vi "Calculator.vi"() -> ()   [LabVIEW 2014]
panel:
  in  ".":bool
  in  "0":bool
  out "display":string
  in  "=":bool
  in  "plus":bool
  in  "clear":bool
  in  "minus":bool
  in  "3":bool
  in  "2":bool
  in  "1":bool
  in  "multiply":bool
  in  "6":bool
  in  "5":bool
  in  "4":bool
  in  "division":bool
  in  "9":bool
  in  "8":bool
  in  "7":bool
  # "Calculator"
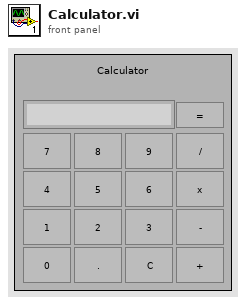
[diagram p1: front panel]
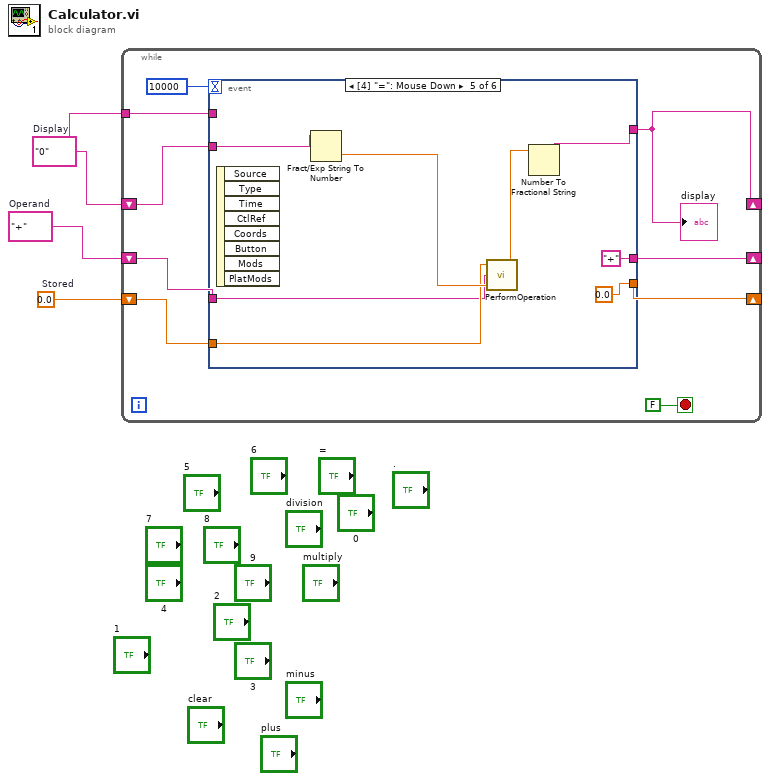
[diagram p0: block diagram]
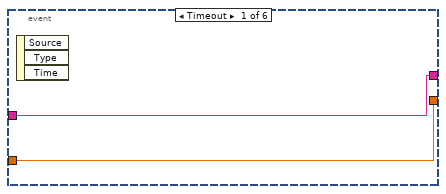
[diagram p2: hidden frame]
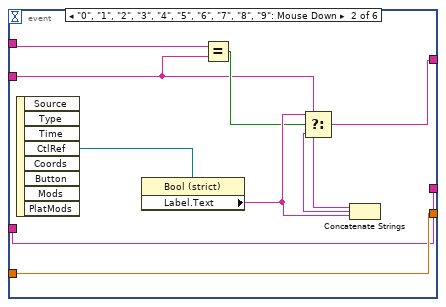
[diagram p3: hidden frame]
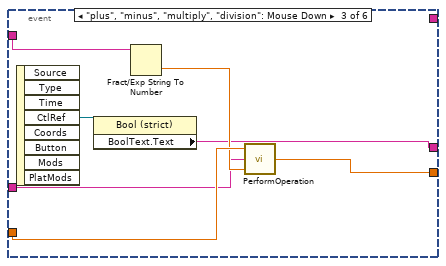
[diagram p4: hidden frame]
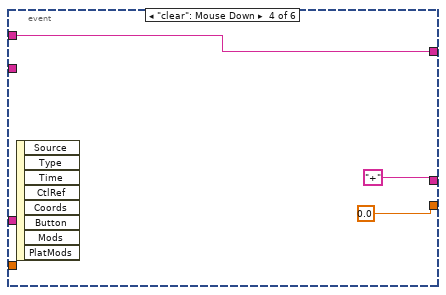
[diagram p5: hidden frame]
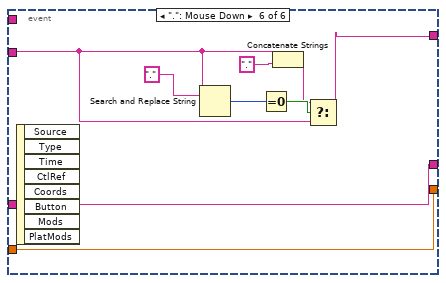
[diagram p6: hidden frame]
diagram:
  w2 = "+"  # Operand
  w1 = 0.0  # Stored
  w3 = "0"  # Display
  n1 = while {
    shift-right: [w8] -> _
    shift-left: w3 -> [w10]
    tunnel: w3 -> [w9]
    shift-right: [w4] -> _
    shift-left: w2 -> [w7]
    shift-right: [w5] -> _
    shift-left: w1 -> [w6]
    stop <- FALSE stop-if-true
    n2 = event shown="[4] \"=\": Mouse Down" {
      selector: _ -> [_ _ _ _ _ _]
      dyn-events: _ -> [_ _ _ _ _ _]
      timeout: 10000 -> [_ _ _ _ _ _]
      tunnel: w10 -> [_ w17 w29 _ w40 w46]
      tunnel: w9 -> [_ w18 _ w33 _ _]
      tunnel: [_ w20 _ w33 w34 w44] -> w8
      tunnel: w7 -> [w14 w15 w27 _ w38 w43]
      tunnel: w6 -> [w13 w16 w30 _ w39 w42]
      tunnel: [w13 w16 w26 0.0 ("Answer") 0.0 ("Answer") w42] -> w5
      tunnel: [w14 w15 w24 "+" ("Label.Text") "+" ("Label.Text") w43] -> w4
      event Timeout {
        n3 = event-data() -> ()  [unwired: 1 in, 3 out]
      }
      event "0", "1", "2", "3", "4", "5", "6", "7", "8", "9": Mouse Down {
        n4 = event-data() -> ("CtlRef"=w23:refnum<vi>)  [unwired: 1 in, 7 out]
        n5 = property class="Bool (strict)"(reference=w23) -> ("Label.Text"=w22:string)  [unwired: 1 in, 2 out]
        n6 = Equal?(x=w18, y=w17) -> (x = y?=w19:bool)
        n7 = Concatenate Strings(w17, w22) -> (w21:string)
        n8 = Select(t=w22, s=w19, f=w21) -> (s? t:f=w20:string)
      }
      event "plus", "minus", "multiply", "division": Mouse Down {
        n9 = event-data() -> ("CtlRef"=w25:refnum<vi>)  [unwired: 1 in, 7 out]
        n10 = property class="Bool (strict)"(reference=w25) -> ("BoolText.Text"=w24:string)  [unwired: 1 in, 2 out]
        n11 = Fract/Exp String To Number(string=w29) -> (number=w28:dbl)  [unwired: 3 in, 1 out]
        n12 = call "PerformOperation.vi"("Operand 2"=w28, "Operation"=w27, "Operand1"=w30) -> ("Answer"=w26:dbl)
      }
      event "clear": Mouse Down {
        n13 = event-data() -> ()  [unwired: 1 in, 8 out]
      }
      event "=": Mouse Down {
        n14 = event-data() -> ()  [unwired: 1 in, 8 out]
        n15 = Fract/Exp String To Number(string=w40) -> (number=w41:dbl)  [unwired: 3 in, 1 out]
        n16 = call "PerformOperation.vi"("Operand 2"=w41, "Operation"=w38, "Operand1"=w39) -> ("Answer"=w35:dbl)
        n17 = Number To Fractional String(number=w35) -> (F-format string=w34:string)  [unwired: 3 in]
      }
      event ".": Mouse Down {
        n18 = event-data() -> ()  [unwired: 1 in, 8 out]
        n19 = Search and Replace String(input string=w46, search string=".") -> (number of replacements=w49:i32)  [unwired: 6 in, 3 out]
        n20 = Equal To 0?(x=w49) -> (x = 0?=w48:bool)
        n21 = Concatenate Strings(w46, "." ("string")) -> (w45:string)
        n22 = Select(t=w45, s=w48, f=w46) -> (s? t:f=w44:string)
      }
    }
    "display" <- w8
  }
